vi "Global Gestione stop se eq termico.vi"() -> ()   [LabVIEW 2019]
panel:
  in  "Tmax raggiunto":bool
  in  "Eq. termico?":bool
  in  "Lettura avvenuta":bool
  in  "Termina dopo misura res":bool
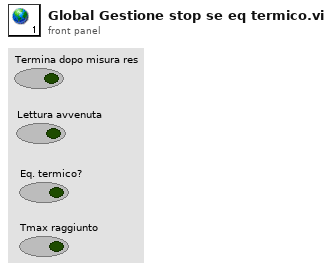
[diagram p1: front panel]
diagram:
